vi "Read Initialized_.vi"(8 "error in (no error)":errorcluster, 11 "navX - Base in":refnum<class "navX - Interface.lvclass">) -> (0 "error out":errorcluster, 2 "Initialized?":bool, 3 "navX - Base out":refnum<class "navX - Interface.lvclass">)   [LabVIEW 2015, in "navX Library v3.lvlib" / "navX - Interface.lvclass"]
uses:
  navX - Interface.lvclass
  navX - Interface.lvclass/navX - Interface.ctl
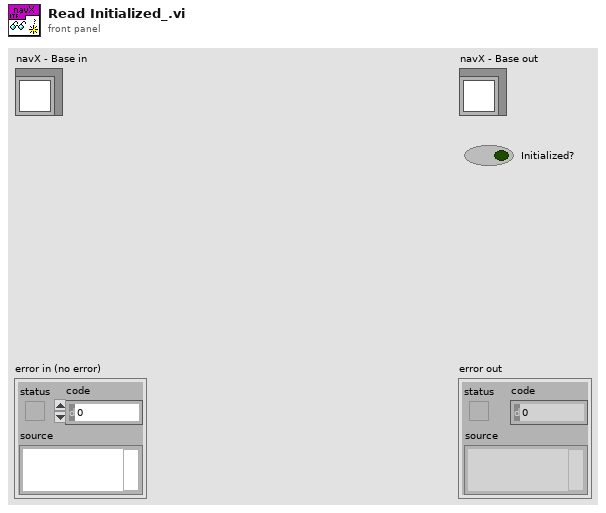
[diagram p1: front panel]
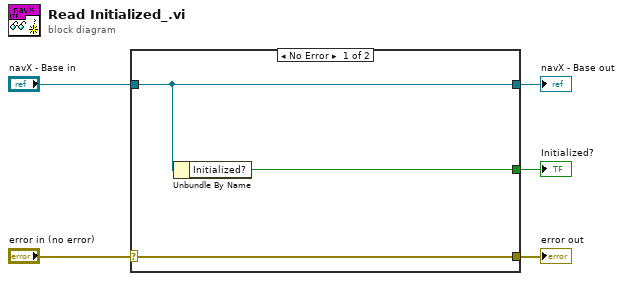
[diagram p0: block diagram]
diagram:
  n1 = case shown="No Error" "error in (no error)" {
    selector: "error in (no error)" -> [w8 w9]
    tunnel: [w8 w9] -> w4
    tunnel: [w7 w10] -> w2
    tunnel: "navX - Base in" -> [w7 w10]
    tunnel: [w6 _] -> w1
    frame No Error {
      n2 = Unbundle By Name(w7) -> ("Initialized?"=w6:bool)
    }
    frame Error {
    }
  }
  "error out" <- w4
  "navX - Base out" <- w2
  "Initialized?" <- w1
